vi "WF_2.vi"() -> ()   [LabVIEW 2013]
uses:
  <vilib>/Utility/error.llb/DialogType.ctl
  <vilib>/DAQmx/write.llb/DAQmx Write (Analog 1D DBL NChan 1Samp).vi
  <vilib>/DAQmx/create/channels.llb/DAQmx Create Channel (AO-Voltage-Basic).vi
  <vilib>/DAQmx/miscellaneous.llb/DAQmx Fill In Error Info.vi
panel:
  in  "Channels":tag[](array[tag])=["cDAQ1Mod1/ao9", "cDAQ1Mod1/ao3", "cDAQ1Mod1/ao5"]
  in  "曝光时间/ms":u32=20
  in  "num":dbl[](array[numeric])=[3.0, 3.0]
  in  "step":dbl[](array[numeric])=[1.36, 1.36]
  in  "start":dbl[](array[numeric])=[-1.5154, -1.4988]
  # "andor 触发"
  # "488"
  # "561"
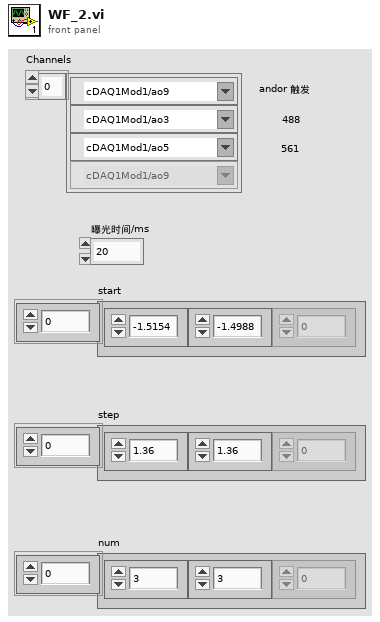
[diagram p1: front panel]
types:
  T1 = typedef "DialogType.ctl" = u16
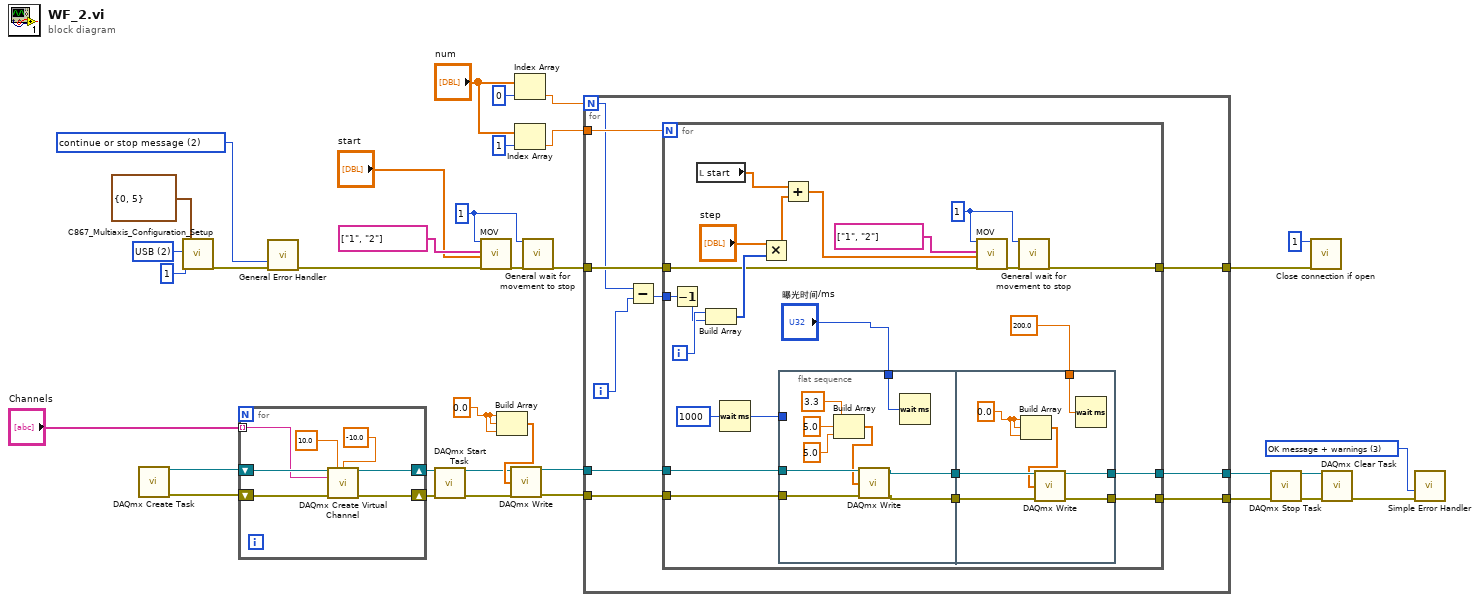
[diagram p0: block diagram]
diagram:
  w6 = 0.0 ("data")
  w14 = T1 3 items=["no dialog", "OK message", "continue or stop message", "OK message + warnings", "continue/stop + warnings"] ("type of dialog (OK msg:1)")
  w22 = 1 ("System no.")
  w26 = T1 2 items=["no dialog", "OK message", "continue or stop message", "OK message + warnings", "continue/stop + warnings"] ("type of dialog (OK msg:1)")
  w30 = u16 2 items=["RS232", "RS232 DaisyChain", "USB"] ("Interface")
  n1 = call <vilib>:"DAQmx Create Task.vi"() -> ("task out"=w8:refnum<k21>, "error out"=w7:errorcluster)  [unwired: 14 in]
  n2 = call "C867_Multiaxis_Configuration_Setup.vi"("System no."=1, "Interface"=w30, "RS232 settings"=cluster{"Portnumber":i32, "Baudrate":u16} {"Portnumber"=0, "Baudrate"=5}) -> ("error out"=w27:errorcluster)  [unwired: 10 in, 6 out]
  n3 = for {
    shift-right: [w40] -> w25
    shift-left: w8 -> [w38]
    shift-right: [w39] -> w24
    shift-left: w7 -> [w37]
    tunnel: "Channels" -> [w36] mode=indexing
    n4 = call-poly <vilib>:"DAQmx Create Virtual Channel.vi"("task in"=w38, "maximum value"=10.0, "minimum value"=-10.0, "physical channels"=w36, "error in"=w37) -> ("task out"=w40:refnum<k21>, "error out"=w39:errorcluster)  [unwired: 9 in]
  }
  n5 = call <vilib>:"General Error Handler.vi"("type of dialog (OK msg:1)"=w26, "error in (no error)"=w27) -> ("error out"=w19:errorcluster)  [unwired: 9 in, 4 out]
  n6 = call <vilib>:"DAQmx Start Task.vi"("task/channels in"=w25, "error in"=w24) -> ("task out"=w4:refnum<k21>, "error out"=w3:errorcluster)  [unwired: 12 in]
  n7 = call "MOV.vi"("System no."=w22, "Axes to move"=string[] ["1", "2"], "Position values"="start", "error in"=w19) -> ("error out"=w23:errorcluster)  [unwired: 15 in]
  n8 = Build Array(w6, w6, w6) -> (w5:dbl[])
  n9 = call-poly <vilib>:"DAQmx Write.vi"("task/channels in"=w4, "data"=w5, "error in"=w3) -> ("task out"=w2:refnum<k21>, "error out"=w1:errorcluster)  [unwired: 10 in, 1 out]
  n10 = Index Array(array="num", index=0) -> (element=w32:dbl)
  n11 = Index Array(array="num", index=1) -> (element=w31:dbl)
  n12 = call "General wait for movement to stop.vi"("System no."=w22, "error in"=w23) -> ("error out"=w18:errorcluster)  [unwired: 16 in, 1 out]
  n13 = for {
    N: w32 -> [w45]
    tunnel: w31 -> [w52]
    tunnel: w18 -> [w51]
    tunnel: w2 -> [w50]
    tunnel: w1 -> [w49]
    tunnel: [w48] -> w13
    tunnel: [w47] -> w12
    tunnel: [w46] -> w10
    i -> [w44]
    n14 = Subtract(x=w45, y=w44) -> (x-y=w43:i32)
    n15 = for {
      N: w52 -> [_]
      tunnel: w51 -> [w70]
      tunnel: w50 -> [w67]
      tunnel: w49 -> [w66]
      tunnel: [w60] -> w48
      tunnel: [w59] -> w47
      tunnel: [w58] -> w46
      tunnel: w43 -> [w56]
      i -> [w57]
      w71 = 1 ("System no.")
      n16 = Decrement(x=w56) -> (x-1=w55:i32)
      n17 = local read "start"() -> (w61:dbl[])
      n18 = Build Array(w57, w55) -> (w74:i32[])
      n19 = Wait (ms)(milliseconds to wait=u32 1000) -> (millisecond timer value=w62:u32)
      n20 = Multiply(x="step", y=w74) -> (x*y=w73:dbl[])
      n21 = flat-sequence {
        tunnel: w67 -> [w84]
        tunnel: w66 -> [w83]
        tunnel: "曝光时间/ms" -> [w82]
        tunnel: [w81] -> w65
        tunnel: [w80] -> w64
        tunnel: w62 -> [_]
        tunnel: w65 -> [w91]
        tunnel: w64 -> [w90]
        tunnel: 200.0 -> [w89]
        tunnel: [w88] -> w60
        tunnel: [w87] -> w59
        frame #0 {
          n22 = Build Array(3.3 ("data"), 5.0, 5.0) -> (w76:dbl[])
          n23 = call-poly <vilib>:"DAQmx Write.vi"("task/channels in"=w84, "data"=w76, "error in"=w83) -> ("task out"=w81:refnum<k21>, "error out"=w80:errorcluster)  [unwired: 10 in, 1 out]
          n24 = Wait (ms)(milliseconds to wait=w82) -> ()  [unwired: 1 out]
        }
        frame #1 {
          w86 = 0.0 ("data")
          n25 = Build Array(w86, w86, w86) -> (w85:dbl[])
          n26 = call-poly <vilib>:"DAQmx Write.vi"("task/channels in"=w91, "data"=w85, "error in"=w90) -> ("task out"=w88:refnum<k21>, "error out"=w87:errorcluster)  [unwired: 10 in, 1 out]
          n27 = Wait (ms)(milliseconds to wait=w89) -> ()  [unwired: 1 out]
        }
      }
      n28 = Add(x=w61, y=w73) -> (x+y=w68:dbl[])
      n29 = call "MOV.vi"("System no."=w71, "Axes to move"=string[] ["1", "2"], "Position values"=w68, "error in"=w70) -> ("error out"=w72:errorcluster)  [unwired: 15 in]
      n30 = call "General wait for movement to stop.vi"("System no."=w71, "error in"=w72) -> ("error out"=w58:errorcluster)  [unwired: 16 in, 1 out]
    }
  }
  n31 = call <vilib>:"DAQmx Stop Task.vi"("task/channels in"=w13, "error in"=w12) -> ("task out"=w16:refnum<k21>, "error out"=w15:errorcluster)  [unwired: 12 in]
  n32 = call "Close connection if open.vi"("System no."=1, "error in"=w10) -> ()  [unwired: 1 in, 17 out]
  n33 = call <vilib>:"DAQmx Clear Task.vi"("task in"=w16, "error in"=w15) -> ("error out"=w17:errorcluster)  [unwired: 13 in]
  n34 = call <vilib>:"Simple Error Handler.vi"("type of dialog (OK msg:1)"=w14, "error in (no error)"=w17) -> ()  [unwired: 3 in, 5 out]
